vi "Discrete Random.vi"   [LabVIEW 2017, in "NI_Gmath.lvlib"]
doc: "Generates random values from a variate X, where X describes the selected distribution type. You must manually select the polymorphic instance to use."
uses:
  <vilib>/gmath/NI_Gmath.lvlib
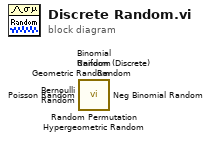
[diagram p0: block diagram]
diagram:
  n1 = call <vilib>:"Random Permutation.vi"() -> ()  [unwired: 10 in, 2 out]
  n2 = call <vilib>:"Uniform (Discrete) Random.vi"() -> ()  [unwired: 10 in, 2 out]
  n3 = call <vilib>:"Poisson Random.vi"() -> ()  [unwired: 10 in, 2 out]
  n4 = call <vilib>:"Neg Binomial Random.vi"() -> ()  [unwired: 10 in, 2 out]
  n5 = call <vilib>:"Hypergeometric Random.vi"() -> ()  [unwired: 10 in, 2 out]
  n6 = call <vilib>:"Geometric Random.vi"() -> ()  [unwired: 10 in, 2 out]
  n7 = call <vilib>:"Binomial Random.vi"() -> ()  [unwired: 10 in, 2 out]
  n8 = call <vilib>:"Bernoulli Random.vi"() -> ()  [unwired: 10 in, 2 out]
